vi "Carbide-Control-Example.vi"() -> ()   [LabVIEW 2014]
doc: "André Romero - 2021\nandretec@ifsc.usp.br\nIFSC - USP"
panel:
  out "N Loops":i32=3
  out "PP Dv Value":dbl=10.0
  in  "PP Divider":dbl=10.0
  out "PP Div value":dbl=1.0
  out "N loops":i32=5
  out "value 2":dbl=10.0
  in  "Value":dbl=10.0
  out "Att value":dbl=86.0
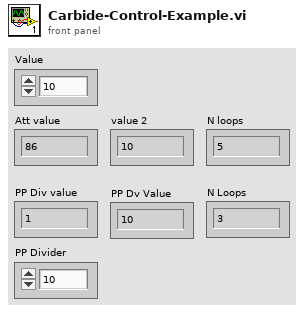
[diagram p1: front panel]
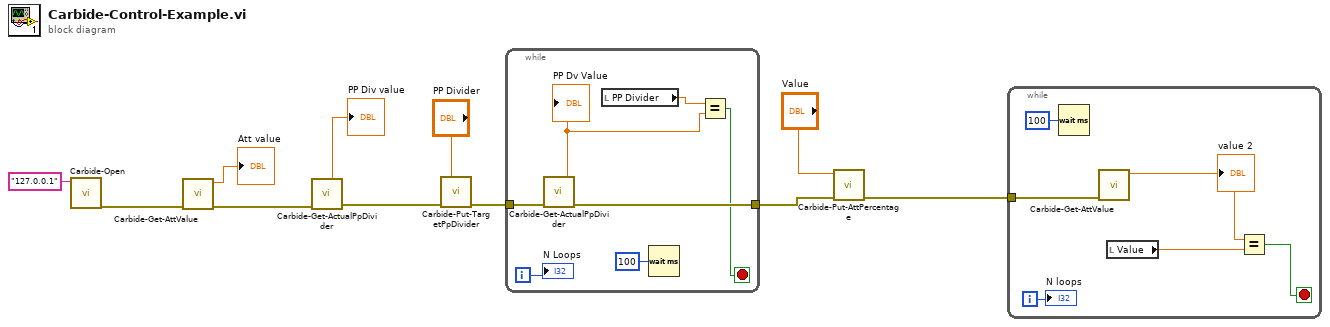
[diagram p0: block diagram]
diagram:
  n1 = call "Carbide-Open.vi"("Laser IP address"="127.0.0.1") -> ("Error Out"=w9:errorcluster)  [unwired: 9 in]
  n2 = call "Carbide-Get-AttValue.vi"("Error In"=w9) -> ("Error Out"=w6:errorcluster, "value"=→"Att value":dbl)  [unwired: 9 in]
  n3 = call "Carbide-Get-ActualPpDivider.vi"("Error In"=w6) -> ("Error Out"=w4:errorcluster, "value"=→"PP Div value":dbl)  [unwired: 9 in]
  n4 = call "Carbide-Put-TargetPpDivider.vi"("Error In"=w4, "Value"="PP Divider") -> ("Error Out"=w2:errorcluster)  [unwired: 9 in]
  n5 = while {
    tunnel: w2 -> [w18]
    tunnel: [w17] -> w1
    i -> [w16]
    stop <- w13 stop-if-true
    n6 = call "Carbide-Get-ActualPpDivider.vi"("Error In"=w18) -> ("Error Out"=w17:errorcluster, "value"=w14:dbl)  [unwired: 9 in]
    "PP Dv Value" <- w14
    n7 = local read "PP Divider"() -> (w15:dbl)
    n8 = Wait (ms)(milliseconds to wait=u32 100) -> ()  [unwired: 1 out]
    n9 = Equal?(x=w15, y=w14) -> (x = y?=w13:bool)
    "N Loops" <- w16
  }
  n10 = call "Carbide-Put-AttPercentage.vi"("Error In"=w1, "Value"="Value") -> ("Error Out"=w7:errorcluster)  [unwired: 9 in]
  n11 = while {
    tunnel: w7 -> [w24]
    i -> [w19]
    stop <- w22 stop-if-true
    n12 = Wait (ms)(milliseconds to wait=u32 100) -> ()  [unwired: 1 out]
    n13 = call "Carbide-Get-AttValue.vi"("Error In"=w24) -> ("value"=w23:dbl)  [unwired: 9 in, 1 out]
    "value 2" <- w23
    n14 = local read "Value"() -> (w20:dbl)
    n15 = Equal?(x=w23, y=w20) -> (x = y?=w22:bool)
    "N loops" <- w19
  }
